vi "总氮插入数据.vi"(0 "table":string, 5 "data":T2={"时间标识"=timestamp(0 s since 1904-01-01), "测量模式"=enum."水样测试", "数据标记表"="N", "监测值"=0.0, "单位"=0, "数据标识"="", "因子编码"=0, "标样参考值"=0.0, "F0"=0.0, "F1"=0.0, "F2"=0.0, "F3"=0.0, "F4"=0.0, "F5"=0.0, "F6"=0.0, "F7"=0.0, "X"=0.0, "温度"=0.0, "湿度"=0.0, "量程标识"="", "SN"=""} {"单位" items=["μg/L", "mg/L", "ppm", "mg/m3", "cm", "ppb", "μg/m3", "%", "nmol/mol", "μmol/mol", "MPN/L", "MPN/100ml", "ng/m3", "NTU", "无量纲", "ms/cm", "μs/cm"]}, 11 "error in (no error)":errorcluster) -> (15 "error out":errorcluster)   [LabVIEW 2016, in "斯坦道总氮.lvlib"]
uses:
  <vilib>/Utility/sysdir.llb/System Directory Type.ctl
  <vilib>/Utility/error.llb/DialogType.ctl
  <vilib>/addons/database/Auxilliary.llb/DB Tools Column Info.ctl
  <vilib>/addons/database/Auxilliary.llb/DB Tools DataTypes.ctl
  <vilib>/addons/database/Connection.llb/DB Tools Open Connec (String).vi
  <vilib>/addons/database/Connection.llb/Conn Execute.vi
  <vilib>/addons/database/Recordset.llb/Rec Fetch Recordset Data (R).vi
  <vilib>/addons/database/Recordset.llb/Rec Destroy - Connection.vi
  <vilib>/addons/database/NI_Database_API.lvlib
panel:
  out "data输出":T1
  out "为空？":bool
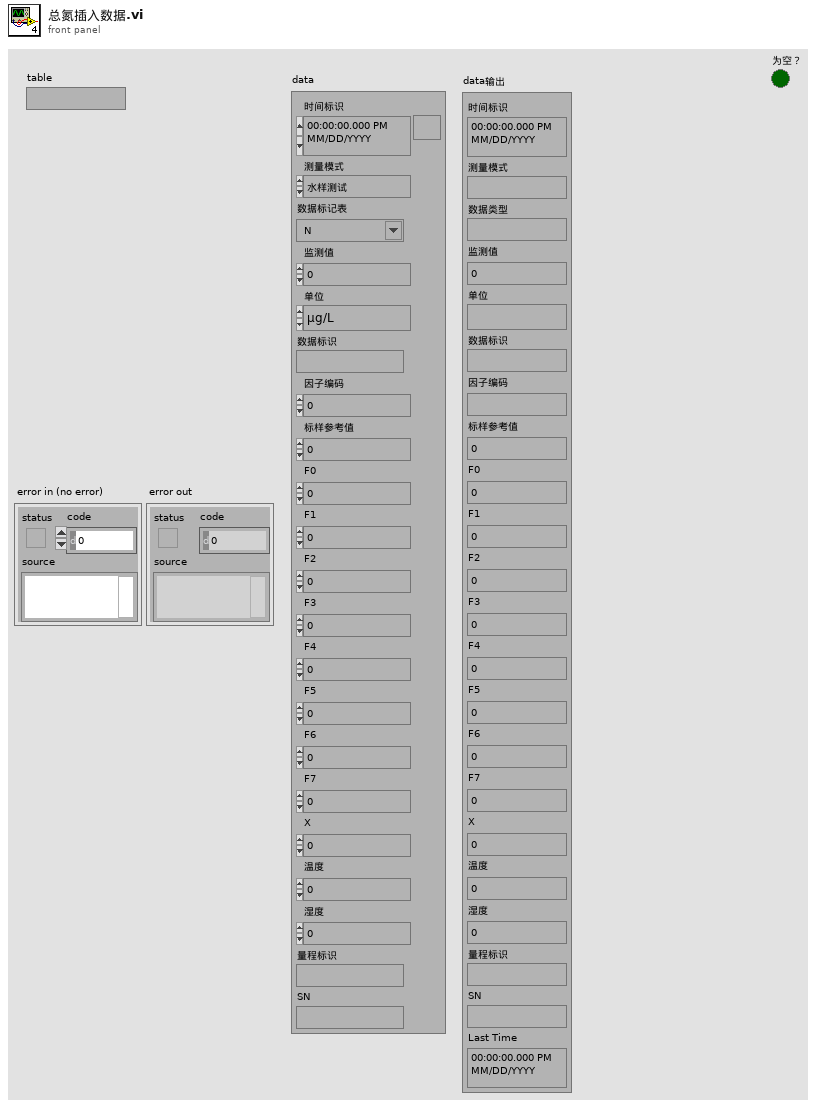
[diagram p1: front panel]
types:
  T1 = cluster{"时间标识":timestamp, "测量模式":string, "数据类型":string, "监测值":sgl, "单位":string, "数据标识":string, "因子编码":string, "标样参考值":sgl, "F0":sgl, "F1":sgl, "F2":sgl, "F3":sgl, "F4":sgl, "F5":sgl, "F6":sgl, "F7":sgl, "X":sgl, "温度":sgl, "湿度":sgl, "量程标识":string, "SN":string, "Last Time":timestamp}
  T2 = cluster{"时间标识":timestamp, "测量模式":enum16{"维护数据", "水样测试", "标样核查", "零点核查", "跨度核查", "空白测试", "平行样测试", "加标回收", "空白校准", "标样校准", "初始化（清洗）"}, "数据标记表":string, "监测值":sgl, "单位":u16, "数据标识":string, "因子编码":u32, "标样参考值":sgl, "F0":sgl, "F1":sgl, "F2":sgl, "F3":sgl, "F4":sgl, "F5":sgl, "F6":sgl, "F7":sgl, "X":sgl, "温度":sgl, "湿度":sgl, "量程标识":string, "SN":string}
  T3 = typedef "DialogType.ctl" = u16
  T4 = typedef "System Directory Type.ctl" = i32
  T5 = typedef "NI_Database_API.lvlib/Conn ObjectReference.ctl" = refnum<k1>
  T6 = typedef "NI_Database_API.lvlib/Rec ObjectReference.ctl" = refnum<k1>
  T7 = typedef "NI_Database_API.lvlib/DB Tools Column Info.ctl" = cluster{"column name":string, "data type":T8, "size":i32, "allow null?":bool}
  T8 = typedef "NI_Database_API.lvlib/DB Tools DataTypes.ctl" = enum16{"String", "Long (I32)", "Single (SGL)", "Double (DBL)", "Date/Time", "Binary"}
  T9 = enum16{"维护数据", "水样测试", "标样核查", "零点核查", "跨度核查", "空白测试", "平行样测试", "加标回收", "空白校准", "标样校准", "初始化（清洗）"}
  T10 = cluster{"测量量程":dbl, "测量精度":dbl, "测量间隔":dbl, "消解温度":dbl, "消解时长":dbl, "空白校准时间":timestamp, "曲线截距":dbl, "曲线斜率":dbl, "测量检出限":dbl, "测量信号值":dbl, "线性相关系数":dbl, "二次多项式系数":dbl, "标样校准时间":timestamp, "稀释倍数":dbl, "三项式系数":dbl, "空白标定系数":dbl, "量程系数":dbl, "F0/ORPA":dbl, "F1/ORPB":dbl, "F2/ORPK":dbl, "F3":dbl, "F4":dbl, "F5":dbl, "F6":dbl, "F7":dbl, "X0/滴定数":dbl, "量程":dbl}
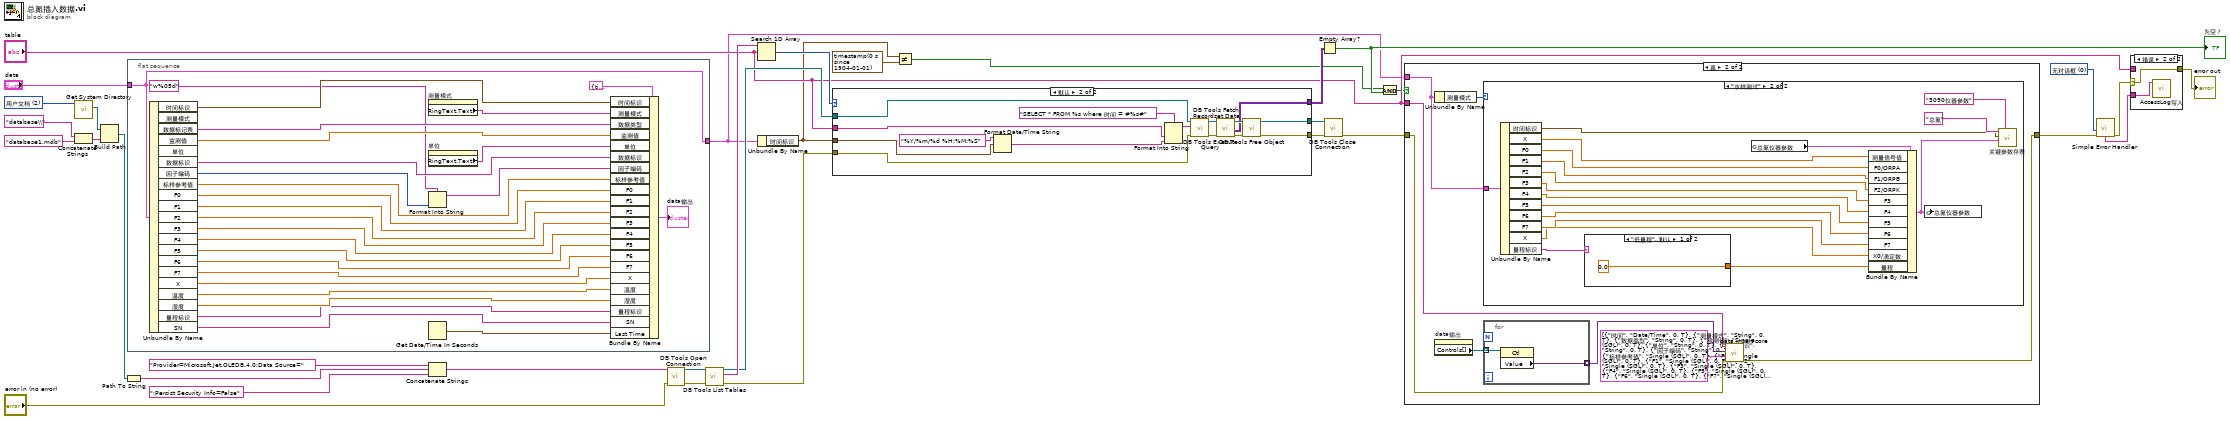
[diagram p0: block diagram]
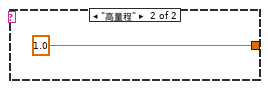
[diagram p5: hidden frame]
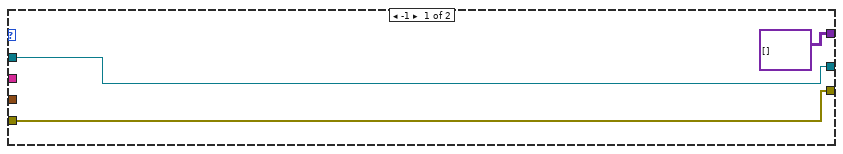
[diagram p6: hidden frame]
diagram:
  w15 = T3 0 items=["无对话框", "确定信息", "继续或停止信息", "确定信息＋警告", "继续/停止+警告"] ("type of dialog (OK msg:1)")
  w33 = T4 2 items=["用户目录"=0, "用户桌面"=1, "用户文档"=2, "用户应用程序数据"=3, "用户设置"=4, "用户临时目录"=5, "公共文档"=6, "公共应用程序数据"=7, "公共设置"=8, "公共缓存"=13, "系统核心库"=9, "系统安装库"=10, "应用程序文件"=11, "启动盘根目录"=12] ("system directory type")
  n1 = call <vilib>:"Get System Directory.vi"("system directory type"=w33) -> ("system directory"=w31:path)  [unwired: 10 in]
  n2 = Concatenate Strings("database\\" ("condition"), "database1.mdb" ("database")) -> (w25:string)
  n3 = Build Path(base path=w31, name or relative path=w25) -> (appended path=w30:path)
  n4 = Path To String(path=w30) -> (string=w29:string)
  n5 = flat-sequence {
    tunnel: "data" -> [w38]
    tunnel: [w38] -> w9
    frame #0 {
      n6 = Unbundle By Name(w38) -> ("时间标识"=w59:timestamp, "数据标记表"=w57:string, "监测值"=w56:sgl, "数据标识"=w54:string, "因子编码"=w37:u32, "标样参考值"=w53:sgl, "F0"=w52:sgl, "F1"=w51:sgl, "F2"=w50:sgl, "F3"=w49:sgl, "F4"=w48:sgl, "F5"=w47:sgl, "F6"=w46:sgl, "F7"=w45:sgl, "X"=w44:sgl, "温度"=w43:sgl, "湿度"=w42:sgl, "量程标识"=w41:string, "SN"=w40:string)  [unwired: 2 out]
      n7 = property on="测量模式" class="Enum (严格)"() -> ("RingText.Text"=w58:string)  [unwired: 2 in, 2 out]
      n8 = property on="单位" class="Ring (严格)"() -> ("RingText.Text"=w55:string)  [unwired: 2 in, 2 out]
      n9 = Format Into String(format string="w%05d" ("格式字符串"), w37) -> (resulting string=w35:string)  [unwired: 2 in, 1 out]
      n10 = Get Date/Time In Seconds() -> (seconds since 1Jan1904=w39:timestamp)
      n11 = Bundle By Name(cluster=T1 {"时间标识"=timestamp(0 s since 1904-01-01), "测量模式"="", "数据类型"="", "监测值"=0.0, "单位"="", "数据标识"="", "因子编码"="", "标样参考值"=0.0, "F0"=0.0, "F1"=0.0, "F2"=0.0, "F3"=0.0, "F4"=0.0, "F5"=0.0, "F6"=0.0, "F7"=0.0, "X"=0.0, "温度"=0.0, "湿度"=0.0, "量程标识"="", "SN"="", "Last Time"=timestamp(0 s since 1904-01-01)} ("data输出"), "时间标识"=w59, "测量模式"=w58, "数据类型"=w57, "监测值"=w56, "单位"=w55, "数据标识"=w54, "因子编码"=w35, "标样参考值"=w53, "F0"=w52, "F1"=w51, "F2"=w50, "F3"=w49, "F4"=w48, "F5"=w47, "F6"=w46, "F7"=w45, "X"=w44, "温度"=w43, "湿度"=w42, "量程标识"=w41, "SN"=w40, "Last Time"=w39) -> (→"data输出":T1)
    }
  }
  n12 = Concatenate Strings("Provider=Microsoft.Jet.OLEDB.4.0;Data Source=" ("condition"), w29, ";Persist Security Info=False" ("condition")) -> (w27:string)
  n13 = call-poly <vilib>:"DB Tools Open Connection.vi"("error in (no error)"="error in (no error)", "connection information"=w27) -> ("error out"=w22:errorcluster, "connection reference"=w23:T5)  [unwired: 6 in]
  n14 = call <vilib>:"DB Tools List Tables.vi"("error in (no error)"=w22, "connection reference"=w23) -> ("error out"=w16:errorcluster, "tables"=w21:string[], "connection reference out"=w17:T5)  [unwired: 3 in]
  n15 = Search 1D Array(1D array=w21, element="table") -> (index of element=w20:i32)  [unwired: 1 in]
  n16 = Unbundle By Name(w9) -> ("时间标识"=w7:timestamp)
  n17 = case shown="默认" w20 {
    tunnel: [variant[][] [] ("recordset data") w75] -> w24
    tunnel: [w64 w74] -> w4
    tunnel: [w63 w73] -> w3
    tunnel: w17 -> [w64 w69]
    tunnel: w16 -> [w63 w68]
    tunnel: "table" -> [_ w67]
    tunnel: w7 -> [_ w65]
    frame -1 {
    }
    frame Default {
      n18 = Format Date/Time String(time format string (%c)="%Y/%m/%d %H:%M:%S" ("时间格式字符串(%c)"), seconds (now)=w65) -> (date/time string=w70:string)  [unwired: 1 in]
      n19 = Format Into String(format string="SELECT * FROM %s where 时间 = #%s#" ("格式字符串"), w67, w70) -> (resulting string=w72:string)  [unwired: 2 in, 1 out]
      n20 = call-poly <vilib>:"DB Tools Execute Query.vi"("error in (no error)"=w68, "SQL query"=w72, "connection reference"=w69) -> ("error out"=w76:errorcluster, "recordset reference"=w79:T6)  [unwired: 5 in]
      n21 = call-poly <vilib>:"DB Tools Fetch Recordset Data.vi"("error in (no error)"=w76, "recordset reference"=w79) -> ("error out"=w77:errorcluster, "recordset data"=w75:variant[][], "recordset reference out"=w78:T6)  [unwired: 3 in]
      n22 = call-poly <vilib>:"DB Tools Free Object.vi"("error in (no error)"=w77, "recordset reference"=w78) -> ("error out"=w73:errorcluster, "connection reference"=w74:T5)  [unwired: 8 in]
    }
  }
  n23 = Not Equal?(x=w7, y=timestamp(0 s since 1904-01-01)) -> (x != y?=w5:bool)
  n24 = Empty Array?(array=w24) -> (empty?=w18:bool)
  "为空？" <- w18
  n25 = call <vilib>:"DB Tools Close Connection.vi"("error in (no error)"=w3, "connection reference"=w4) -> ("error out"=w2:errorcluster)  [unwired: 5 in]
  n26 = And(x=w5, y=w18) -> (x .and. y?=w6:bool)
  n27 = case shown="真" w6 {
    tunnel: "table" -> [_ w85]
    tunnel: w9 -> [_ w82]
    tunnel: w2 -> [w80 w83]
    tunnel: [w80 w84] -> w1
    frame False {
    }
    frame True {
      n28 = Unbundle By Name(w82) -> ("测量模式"=w81:T9)
      n29 = property on="data输出" class="Clust (严格)"() -> ("Controls[]"=w86:refnum<vi>[])  [unwired: 2 in, 2 out]
      n30 = case shown="\"水样测试\"" w81 {
        tunnel: w82 -> [_ w105]
        frame "维护数据", Default {
        }
        frame "水样测试" {
          n31 = Unbundle By Name(w105) -> ("时间标识"=w104:timestamp, "X"=w103:sgl, "F0"=w101:sgl, "F1"=w100:sgl, "F2"=w99:sgl, "F3"=w98:sgl, "F4"=w97:sgl, "F5"=w96:sgl, "F6"=w95:sgl, "F7"=w94:sgl, "X"=w93:sgl, "量程标识"=w92:string)
          n32 = case shown="\"低量程\", 默认" w92 {
            tunnel: [0.0 1.0] -> w91
            frame "低量程", Default {
            }
            frame "高量程" {
            }
          }
          n33 = global read "总氮断电保存全局变量.vi" "总氮仪器参数"() -> (w108:T10)
          n34 = Bundle By Name(cluster=w108, "测量信号值"=w103, "F0/ORPA"=w101, "F1/ORPB"=w100, "F2/ORPK"=w99, "F3"=w98, "F4"=w97, "F5"=w96, "F6"=w95, "F7"=w94, "X0/滴定数"=w93, "量程"=w91) -> (w107:T10)
          n35 = global write "总氮断电保存全局变量.vi" "总氮仪器参数"(w107) -> ()
          n36 = call "关键参数存表.vi"("table"="3090仪器参数", "仪器参数"=w107, "datatime"=w104, "仪器名称"="总氮") -> ()  [unwired: 7 in, 1 out]
        }
      }
      n37 = for {
        tunnel: w86 -> [w90] mode=indexing
        tunnel: [w89] -> w88 mode=indexing
        n38 = property class="Ctl"(reference=w90) -> ("Value"=w89:variant)  [unwired: 1 in, 2 out]
      }
      n39 = call "data insert core.vi"("error in (no error)"=w83, "column information"=T7[] [{"column name"="时间", "data type"=enum."Date/Time", "size"=0, "allow null?"=TRUE}, {"column name"="测量模式", "data type"=enum."String", "size"=0, "allow null?"=TRUE}, {"column name"="数据类型", "data type"=enum."String", "size"=0, "allow null?"=TRUE}, {"column name"="检测值", "data type"=enum."Single (SGL)", "size"=0, "allow null?"=TRUE}, {"column name"="单位", "data type"=enum."String", "size"=0, "allow null?"=TRUE}, {"column name"="数据标识", "data type"=enum."String", "size"=0, "allow null?"=TRUE}, {"column name"="因子编码", "data type"=enum."String", "size"=0, "allow null?"=TRUE}, {"column name"="标样参考值", "data type"=enum."Single (SGL)", "size"=0, "allow null?"=TRUE}, {"column name"="F0", "data type"=enum."Single (SGL)", "size"=0, "allow null?"=TRUE}, {"column name"="F1", "data type"=enum."Single (SGL)", "size"=0, "allow null?"=TRUE}, {"column name"="F2", "data type"=enum."Single (SGL)", "size"=0, "allow null?"=TRUE}, {"column name"="F3", "data type"=enum."Single (SGL)", "size"=0, "allow null?"=TRUE}, {"column name"="F4", "data type"=enum."Single (SGL)", "size"=0, "allow null?"=TRUE}, {"column name"="F5", "data type"=enum."Single (SGL)", "size"=0, "allow null?"=TRUE}, {"column name"="F6", "data type"=enum."Single (SGL)", "size"=0, "allow null?"=TRUE}, {"column name"="F7", "data type"=enum."Single (SGL)", "size"=0, "allow null?"=TRUE}, {"column name"="X", "data type"=enum."Single (SGL)", "size"=0, "allow null?"=TRUE}, {"column name"="温度", "data type"=enum."Single (SGL)", "size"=0, "allow null?"=TRUE}, {"column name"="湿度", "data type"=enum."Single (SGL)", "size"=0, "allow null?"=TRUE}, {"column name"="量程标识", "data type"=enum."String", "size"=0, "allow null?"=TRUE}, {"column name"="SN", "data type"=enum."String", "size"=0, "allow null?"=TRUE}, {"column name"="LastTime", "data type"=enum."Date/Time", "size"=0, "allow null?"=TRUE}], "data"=w88, "table"=w85) -> ("error out"=w84:errorcluster)  [unwired: 7 in]
    }
  }
  n40 = call <vilib>:"Simple Error Handler.vi"("type of dialog (OK msg:1)"=w15, "error in (no error)"=w1) -> ("error out"=w14:errorcluster, "message"=w13:string)  [unwired: 3 in, 3 out]
  n41 = case shown="错误" w14 {
    selector: w14 -> [_ w111]
    tunnel: w13 -> [_ w112]
    tunnel: "table" -> [_ _]
    tunnel: [_ w111] -> w11
    frame No Error {
    }
    frame Error {
      n42 = call "AccessLog写入.vi"("Log"=w112) -> ()  [unwired: 11 in]
    }
  }
  "error out" <- w11
